vi "testFlushTelFromDds.vi"(8 "error in (no error)":errorcluster) -> (0 "error out":errorcluster)   [LabVIEW 2018]
doc: "Test the flushTel.vi with queueTelFromDds option."
uses:
  src/TcpServer/TcpServer.lvclass
  src/TcpServer/TcpServer.lvclass/TcpServer.ctl
  src/TcpServerTel/TcpServerTel.lvclass/TcpServerTel.ctl
  <vilib>/addons/_JKI Toolkits/Caraya/classes/Assert/Assert Equal Value_Variant.vi
  src/TcpServerTel/TcpServerTel.lvclass
  <vilib>/addons/_JKI Toolkits/Caraya/classes/Test/Test.lvclass
  <vilib>/addons/_JKI Toolkits/Caraya/classes/Assert/Assert.lvclass
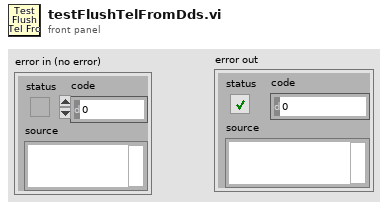
[diagram p1: front panel]
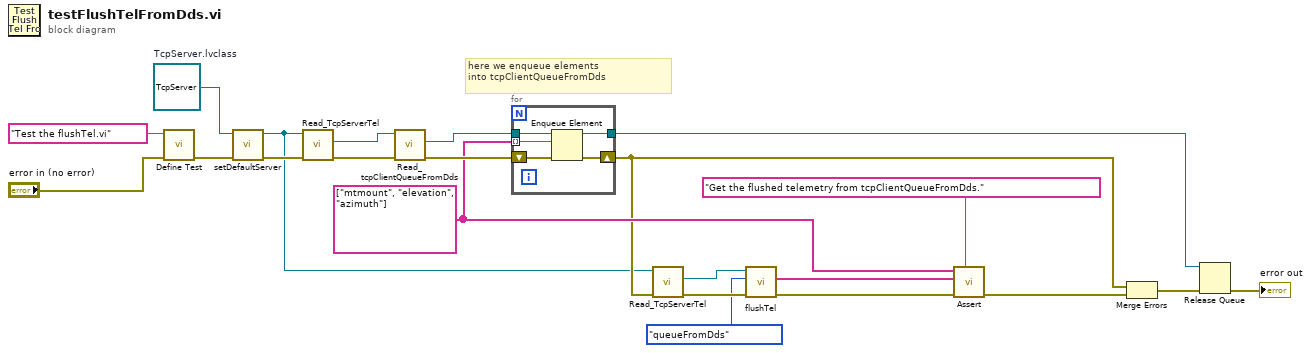
[diagram p0: block diagram]
diagram:
  w7 = string[] ["mtmount", "elevation", "azimuth"]
  w3 = refnum<class "TcpServer.lvclass"> refnum  # TcpServer.lvclass
  # "here we enqueue elements\ninto tcpClientQueueFromDds"
  n1 = call <vilib>:"Define Test.vi"("error in (no error)"="error in (no error)", "Label (VI Title)"="Test the flushTel.vi") -> ("error out"=w21:errorcluster)  [unwired: 9 in]
  n2 = call "setDefaultServer.vi"("error in (no error)"=w21, "TcpServer.lvclass"=w3) -> ("error out"=w10:errorcluster, "tcpServer out"=w2:refnum<class "TcpServer.lvclass">)  [unwired: 8 in]
  n3 = call "Read_TcpServerTel.vi"("error in (no error)"=w10, "TcpServer in"=w2) -> ("error out"=w16:errorcluster, "TcpServerTel.lvclass"=w17:refnum<class "TcpServerTel.lvclass">)  [unwired: 7 in, 1 out]
  n4 = call "Read_tcpClientQueueFromDds.vi"("error in (no error)"=w16, "TcpServerTel in"=w17) -> ("error out"=w13:errorcluster, "tcpClientQueueFromDds"=w12:refnum<queue>)  [unwired: 7 in, 1 out]
  n5 = for {
    tunnel: w12 -> [w26]
    tunnel: w7 -> [w25] mode=indexing
    tunnel: [w23] -> w11
    shift-right: [w24] -> w6
    shift-left: w13 -> [w27]
    n6 = Enqueue Element(queue=w26, element=w25, error in (no error)=w27) -> (queue out=w23:refnum<queue>, error out=w24:errorcluster)  [unwired: 1 in, 1 out]
  }
  n7 = call "Read_TcpServerTel.vi"("error in (no error)"=w6, "TcpServer in"=w2) -> ("error out"=w5:errorcluster, "TcpServerTel.lvclass"=w4:refnum<class "TcpServerTel.lvclass">)  [unwired: 7 in, 1 out]
  n8 = call "flushTel.vi"("error in (no error)"=w5, "queueName"=enum16{"queueFromDds", "queueToDds"}."queueFromDds", "tcpServerTel in"=w4) -> ("error out"=w9:errorcluster, "telemetry flushed"=w8:string[])  [unwired: 6 in, 1 out]
  n9 = call-poly <vilib>:"Assert.vi"("Label"="Get the flushed telemetry from tcpClientQueueFromDds.", "error in (no error)"=w9, "Y"=w8, "X"=w7) -> ("error out"=w18:errorcluster)  [unwired: 7 in]
  n10 = Merge Errors(w6, w18) -> (w14:errorcluster)
  n11 = Release Queue(queue=w11, error in (no error)=w14) -> (error out=→"error out":errorcluster)  [unwired: 1 in, 2 out]
